vi "Add Numeric Comparators.vi"(10 "Comparison":string, 11 "Array in":string[](array[string])) -> (3 "Array out":string[](array[string]))   [LabVIEW 2020, in "Astemes_CSVReportPlugin.lvlib" / "TestStand Result Handler.lvclass"]
uses:
  TestStand Result Handler.lvclass
  Columns.ctl
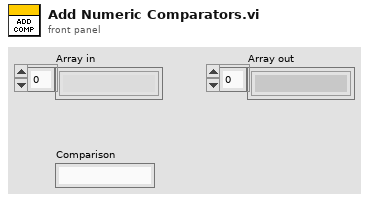
[diagram p1: front panel]
types:
  T1 = typedef "Astemes_CSVReportPlugin.lvlib/TestStand Result Handler.lvclass/Columns.ctl" = enum16{"StepName", "Result", "LowerLimit", "ComparisonTypeLow", "Measurement", "ComparisonTypeHigh", "UpperLimit", "ReportText", "StepType"}
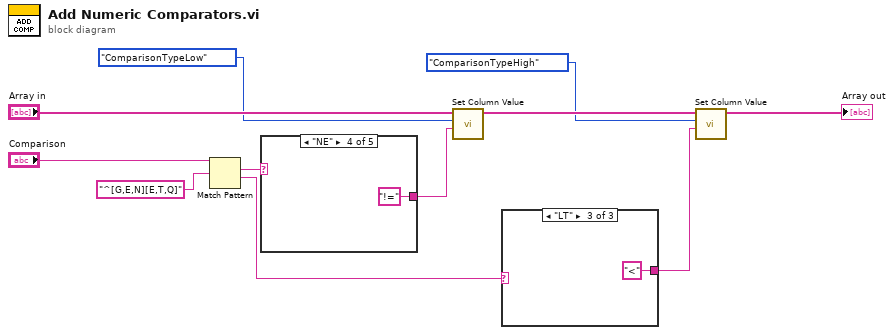
[diagram p0: block diagram]
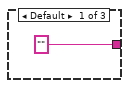
[diagram p2: hidden frame]
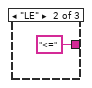
[diagram p3: hidden frame]
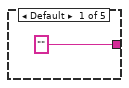
[diagram p4: hidden frame]
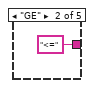
[diagram p5: hidden frame]
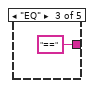
[diagram p6: hidden frame]
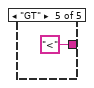
[diagram p7: hidden frame]
diagram:
  n1 = Match Pattern(string="Comparison", regular expression="^[G,E,N][E,T,Q]") -> (match substring=w8:string, after substring=w1:string)  [unwired: 1 in, 2 out]
  n2 = case shown="\"NE\"" w8 {
    tunnel: ["" ("Value") "<=" ("Value") "==" ("Value") "!=" ("Value") "<" ("Value")] -> w7
    frame Default {
    }
    frame "GE" {
    }
    frame "EQ" {
    }
    frame "NE" {
    }
    frame "GT" {
    }
  }
  n3 = call "Set Column Value.vi"("Value"=w7, "Column"=Columns."ComparisonTypeLow", "Empty Row"="Array in") -> ("Array"=w5:string[])  [unwired: 8 in]
  n4 = case shown="\"LT\"" w1 {
    tunnel: ["" ("Value") "<=" ("Value") "<" ("Value")] -> w2
    frame Default {
    }
    frame "LE" {
    }
    frame "LT" {
    }
  }
  n5 = call "Set Column Value.vi"("Value"=w2, "Column"=Columns."ComparisonTypeHigh", "Empty Row"=w5) -> ("Array"=→"Array out":string[])  [unwired: 8 in]
